vi "Disdrometer_SortPlotData.vi"(9 "Plot Data":T1, 10 "Spectrum":dbl[](array[numeric]), 11 "Time, Rate, Accum":dbl[](array[numeric])) -> (1 "Velocity":cluster{dbl[], "Diameter Distribution":dbl[]}(graph), 2 "Size":cluster{dbl[], "Diameter Distribution":dbl[]}(graph), 3 "Observed":dbl, 4 "Rain Rate":cluster{"Today":dbl[], "Today":dbl[]}(graph), 5 "Plot out":T1, 6 "Accumulation":cluster{"Today":dbl[], "Today":dbl[]}(graph))   [LabVIEW 2018]
uses:
  Disdrometer_PlotData_Clust.ctl
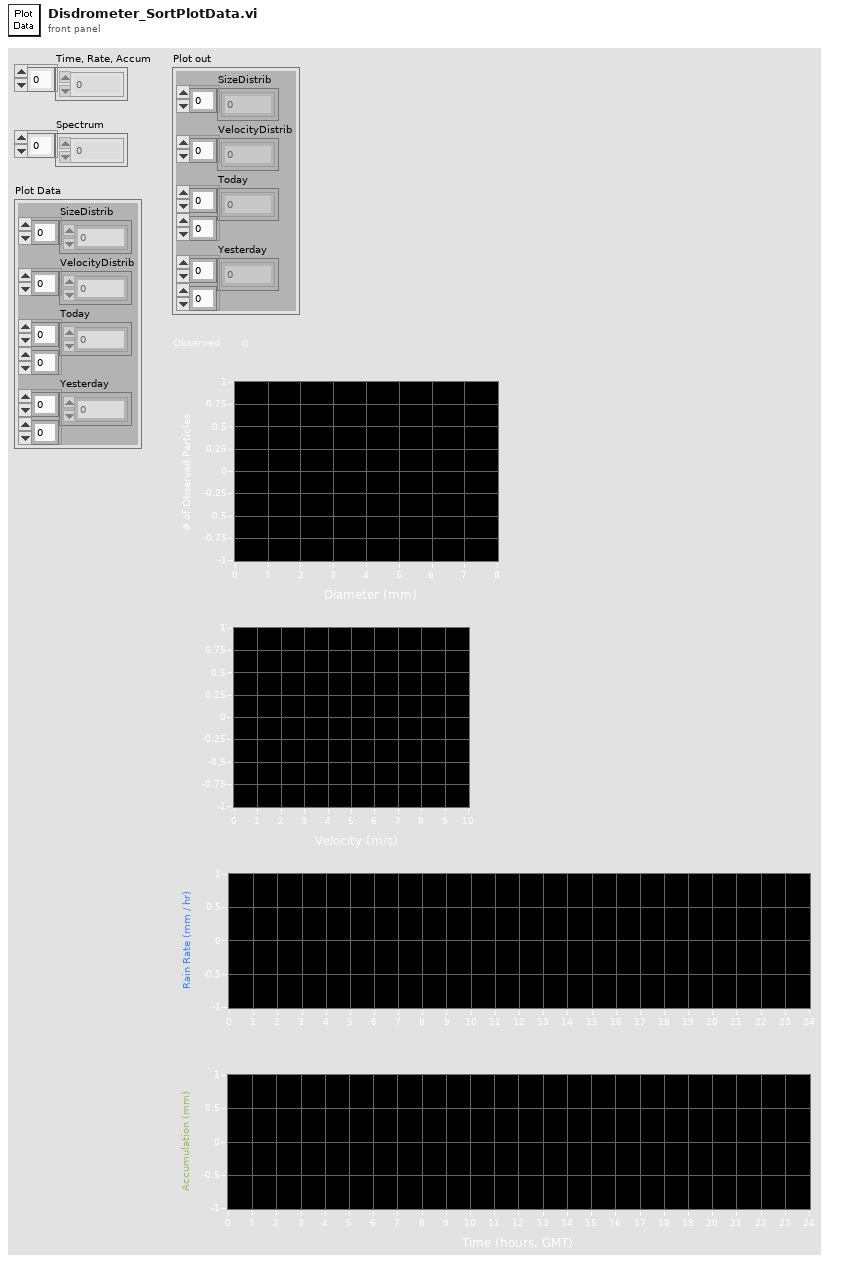
[diagram p1: front panel]
types:
  T1 = typedef "Disdrometer_PlotData_Clust.ctl" = cluster{"SizeDistrib":dbl[], "VelocityDistrib":dbl[], "Today":dbl[][], "Yesterday":dbl[][]}
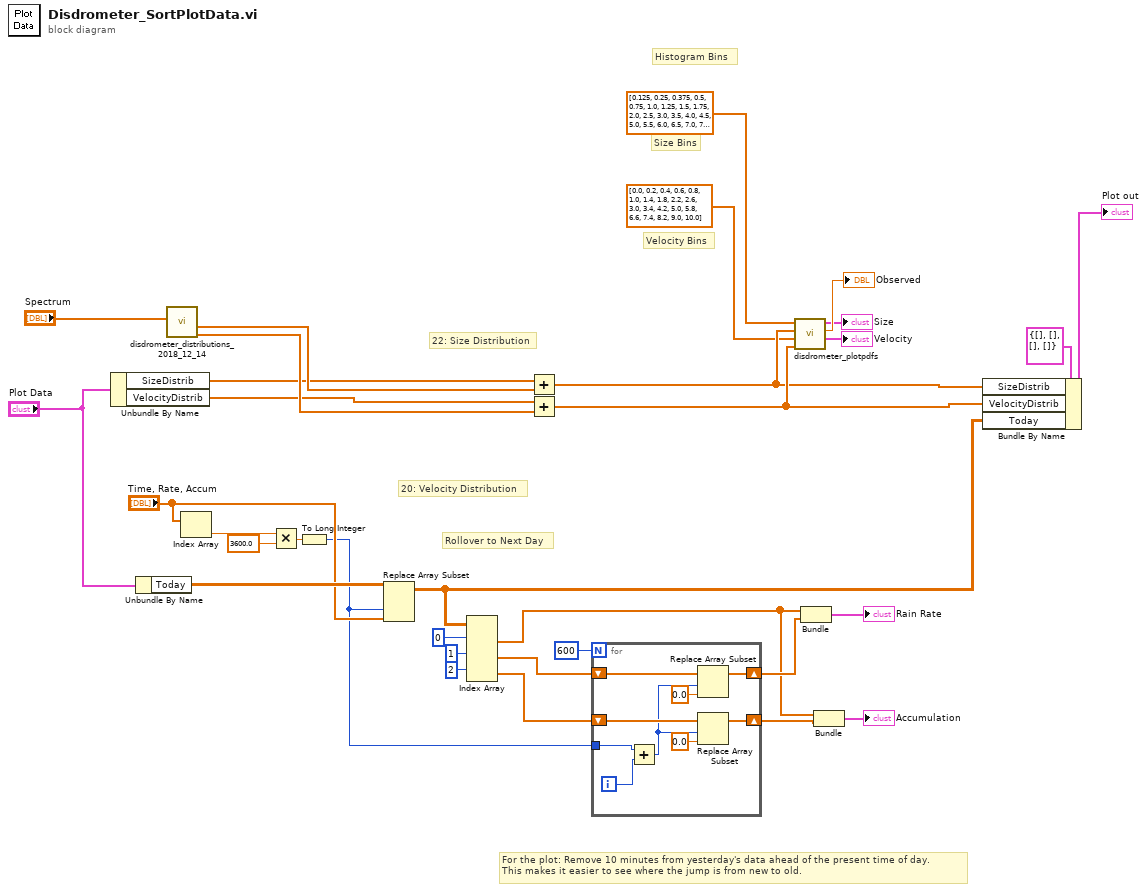
[diagram p0: block diagram]
diagram:
  # "For the plot: Remove 10 minutes from yesterday's data ahead of the present time of day.\nThis makes it easier to see where the jump is from new to old."
  # "Rollover to Next Day"
  # "Histogram Bins"
  # "20: Velocity Distribution"
  # "22: Size Distribution"
  # "Velocity Bins"
  # "Size Bins"
  n1 = Unbundle By Name("Plot Data") -> ("SizeDistrib"=w20:dbl[], "VelocityDistrib"=w19:dbl[])
  n2 = Unbundle By Name("Plot Data") -> ("Today"=w16:dbl[][])
  n3 = call "disdrometer_distributions_2018_12_14.vi"("Spectrum Vector"="Spectrum") -> ("Velocity Distribution"=w23:dbl[], "Diameter Distribution"=w24:dbl[])  [unwired: 8 in, 1 out]
  n4 = Index Array(array="Time, Rate, Accum") -> (element=w18:dbl)  [unwired: 1 in]
  n5 = Multiply(x=w18, y=3600.0) -> (x*y=w14:dbl)
  n6 = To Long Integer(number=w14) -> (32bit integer=w9:i32)
  n7 = Replace Array Subset(array=w16, new element="Time, Rate, Accum", index (col)=w9) -> (w13:dbl[][])  [unwired: 1 in]
  n8 = Index Array(array=w13, index (row) #1=0 ("index (row)"), index (row) #2=1 ("index (row)"), index (row) #3=2 ("index (row)")) -> (element #1=w3:dbl[], element #2=w6:dbl[], element #3=w7:dbl[])  [unwired: 3 in]
  n9 = Add(x=w20, y=w24) -> (x+y=w32:dbl[])
  n10 = Add(x=w19, y=w23) -> (x+y=w33:dbl[])
  n11 = for {
    N: 600 -> [_]
    tunnel: w9 -> [w42]
    shift-right: [w39] -> w4
    shift-left: w7 -> [w40]
    shift-right: [w35] -> w5
    shift-left: w6 -> [w36]
    i -> [w41]
    n12 = Add(x=w42, y=w41) -> (x+y=w34:i32)
    n13 = Replace Array Subset(array=w36, new element=0.0 ("new element/subarray"), index=w34) -> (w35:dbl[])
    n14 = Replace Array Subset(array=w40, new element=0.0 ("new element/subarray"), index=w34) -> (w39:dbl[])
  }
  n15 = call "disdrometer_plotpdfs.vi"("Data B"=w33, "Bins B"=dbl[] [0.0, 0.2, 0.4, 0.6, 0.8, 1.0, 1.4, 1.8, 2.2, 2.6, 3.0, 3.4, 4.2, 5.0, 5.8, 6.6, 7.4, 8.2, 9.0, 10.0], "Data A"=w32, "Bins A"=dbl[] [0.125, 0.25, 0.375, 0.5, 0.75, 1.0, 1.25, 1.5, 1.75, 2.0, 2.5, 3.0, 3.5, 4.0, 4.5, 5.0, 5.5, 6.0, 6.5, 7.0, 7.5, 8.0]) -> ("PDF B"=→"Velocity":cluster{dbl[], dbl[]}, "Na"=→"Observed":dbl, "PDF A"=→"Size":cluster{dbl[], dbl[]})  [unwired: 4 in, 1 out]
  n16 = Bundle("Today"=w3, "Today"=w5) -> (→"Rain Rate":cluster{"Today":dbl[], "Today":dbl[]})  [unwired: 1 in]
  n17 = Bundle("Today"=w3, "Today"=w4) -> (→"Accumulation":cluster{"Today":dbl[], "Today":dbl[]})  [unwired: 1 in]
  n18 = Bundle By Name(cluster=T1 {"SizeDistrib"=[], "VelocityDistrib"=[], "Today"=[], "Yesterday"=[]} ("Plot"), "SizeDistrib"=w32, "VelocityDistrib"=w33, "Today"=w13) -> (→"Plot out":T1)
